vi "test_Task Actor1.vi"() -> ()   [LabVIEW 2023]
uses:
  <vilib>/ActorFramework/Actor/Actor.lvclass
  Task Actor/Task Actor.lvclass
  Task Base/Task Base.lvclass
  Measure and Stimulus Subsystems/Measure and Stimulus Subsystems.lvclass
  ITask Actor/ITask Actor Messages/Perform Action Msg/Perform Action Msg.lvclass
  <vilib>/ActorFramework/Stop Msg/Stop Msg.lvclass
  C:/Program Files/National Instruments/LabVIEW 2023/vi.lib/ActorFramework/Actor/Actor.lvclass
  D:/git/HAL/HAL GOOP4/Task Actor/Task Actor/Task Actor/Task Actor.lvclass
  D:/git/HAL/HAL GOOP4/Task Actor/ITask Actor/ITask Actor/ITask Actor.lvclass
panel:
  out "Waveform Graph Lossy":waveform(dbl)(graph)
  in  "Stop":bool
  in  "Perform Action":bool
  out "error out":errorcluster
  in  "Error in":errorcluster
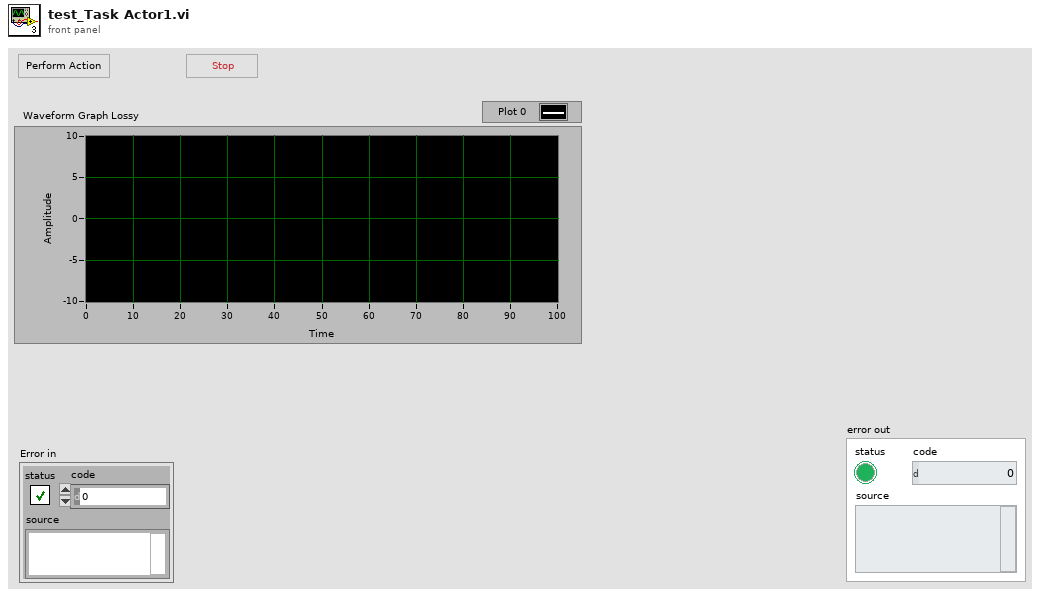
[diagram p1: front panel]
types:
  T1 = cluster{"Stop":refnum<notifier>, "Data":refnum<notifier>}
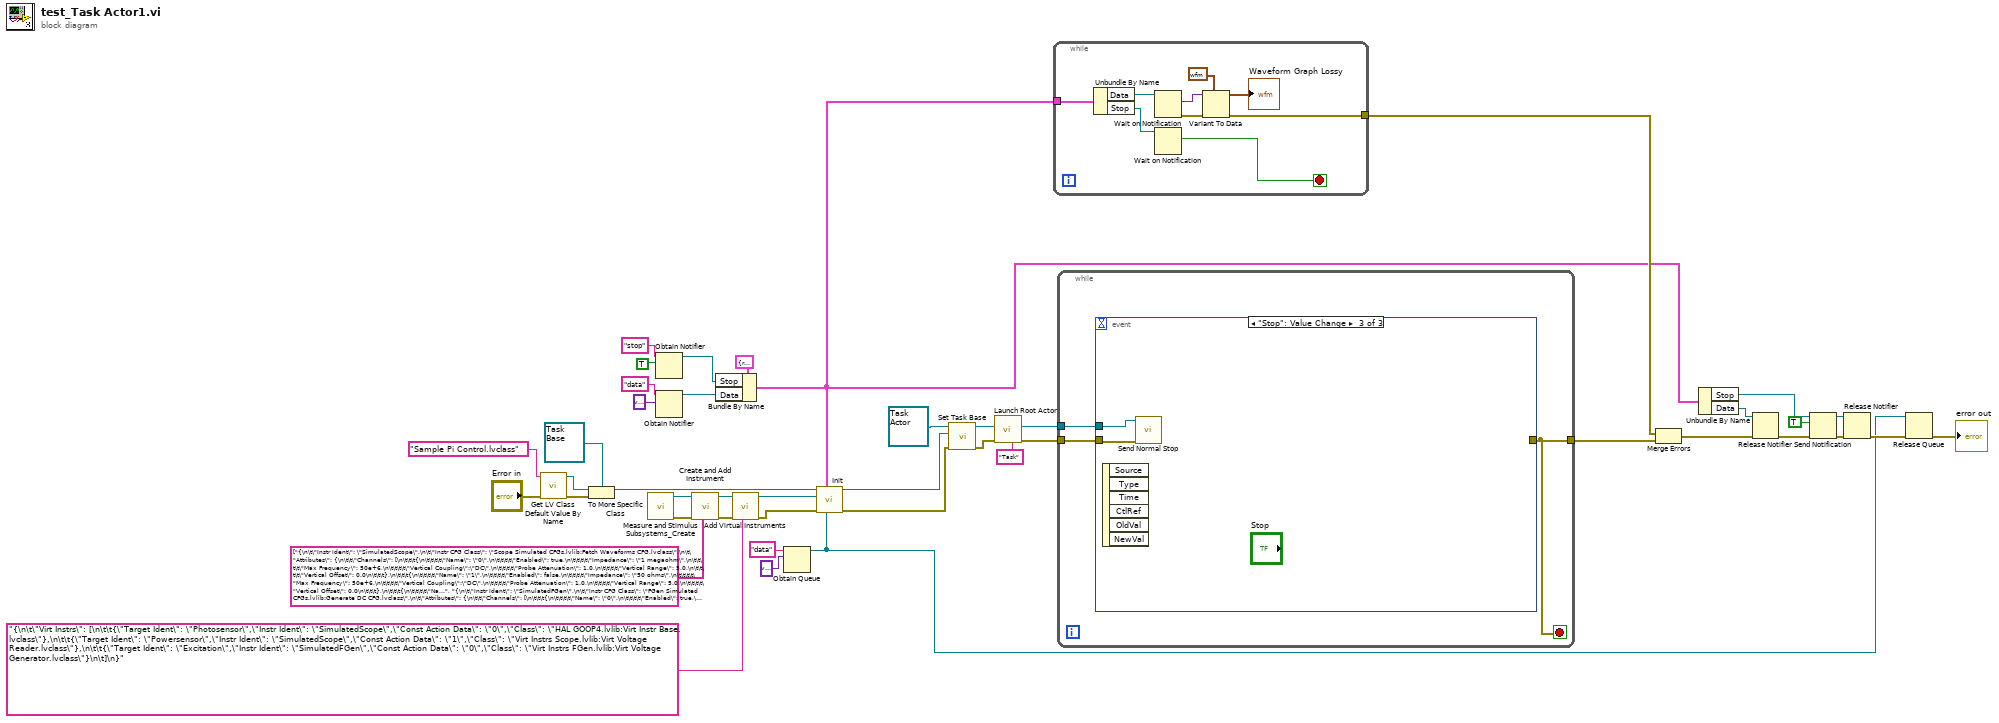
[diagram p0: block diagram]
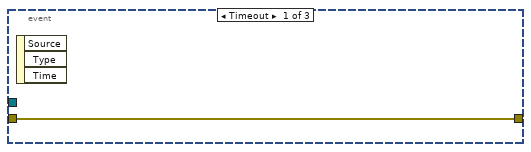
[diagram p2: hidden frame]
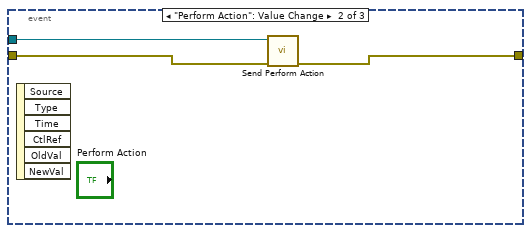
[diagram p3: hidden frame]
diagram:
  n1 = call <vilib>:"Get LV Class Default Value By Name.vi"("error in (no error)"="Error in", "class name"="Sample Pi Control.lvclass") -> ("error out"=w38:errorcluster, "object"=w39:refnum<class>)  [unwired: 8 in]
  n2 = To More Specific Class(target class=refnum<class "Task Base.lvclass"> refnum ("HAL GOOP4.lvlib:Task Base.lvclass"), reference=w39, error in=w38) -> (specific class reference=w36:refnum<class "Task Base.lvclass">)  [unwired: 1 out]
  n3 = call "Measure and Stimulus Subsystems_Create.vi"() -> ("Error Out"=w35:errorcluster, "reference out"=w28:refnum<class "Measure and Stimulus Subsystems.lvclass">)  [unwired: 10 in]
  n4 = Obtain Notifier(name (unnamed)="stop", notification data type=TRUE) -> (notifier out=w23:refnum<notifier>)  [unwired: 2 in, 2 out]
  n5 = Obtain Notifier(name (unnamed)="data", notification data type=variant) -> (notifier out=w22:refnum<notifier>)  [unwired: 2 in, 2 out]
  n6 = call "Create and Add Instrument.vi"("Physical Intr Configs"=string[] ["{\n\t\"Instr Ident\": \"SimulatedScope\",\n\t\"Instr CFG Class\": \"Scope Simulated CFGs.lvlib:Fetch Waveforms CFG.lvclass\",\n\t\"Attributes\": {\n\t\t\"Channels\": [\n\t\t\t{\n\t\t\t\t\"Name\": \"0\",\n\t\t\t\t\"Enabled\": true,\n\t\t\t\t\"Impedance\": \"1 megaohm\",\n\t\t\t\t\"Max Frequency\": 50e+6,\n\t\t\t\t\"Vertical Coupling\":\"DC\",\n\t\t\t\t\"Probe Attenuation\": 1.0,\n\t\t\t\t\"Vertical Range\": 5.0,\n\t\t\t\t\"Vertical Offset\": 0.0\n\t\t\t},\n\t\t\t{\n\t\t\t\t\"Name\": \"1\",\n\t\t\t\t\"Enabled\": false,\n\t\t\t\t\"Impedance\": \"50 ohms\",\n\t\t\t\t\"Max Frequency\": 50e+6,\n\t\t\t\t\"Vertical Coupling\":\"DC\",\n\t\t\t\t\"Probe Attenuation\": 1.0,\n\t\t\t\t\"Vertical Range\": 5.0,\n\t\t\t\t\"Vertical Offset\": 0.0\n\t\t\t},\n\t\t\t{\n\t\t\t\t\"Name\": \"2\",\n\t\t\t\t\"Enabled\": false,\n\t\t\t\t\"Impedance\": \"50 ohms\",\n\t\t\t\t\"Max Frequency\": 50e+6,\n\t\t\t\t\"Vertical Coupling\":\"DC\",\n\t\t\t\t\"Probe Attenuation\": 1.0,\n\t\t\t\t\"Vertical Range\": 5.0,\n\t\t\t\t\"Vertical Offset\": 0.0\n\t\t\t},\n\t\t\t{\n\t\t\t\t\"Name\": \"3\",\n\t\t\t\t\"Enabled\": true,\n\t\t\t\t\"Impedance\": \"50 ohms\",\n\t\t\t\t\"Max Frequency\": 50e+6,\n\t\t\t\t\"Vertical Coupling\":\"DC\",\n\t\t\t\t\"Probe Attenuation\": 1.0,\n\t\t\t\t\"Vertical Range\": 1.4,\n\t\t\t\t\"Vertical Offset\": 0.0\n\t\t\t},\n\t\t\t{\n\t\t\t\t\"Name\": \"4\",\n\t\t\t\t\"Enabled\": false,\n\t\t\t\t\"Impedance\": \"50 ohms\",\n\t\t\t\t\"Max Frequency\": 50e+6,\n\t\t\t\t\"Vertical Coupling\":\"DC\",\n\t\t\t\t\"Probe Attenuation\": 1.0,\n\t\t\t\t\"Vertical Range\": 5.0,\n\t\t\t\t\"Vertical Offset\": 0.0\n\t\t\t},\n\t\t\t{\n\t\t\t\t\"Name\": \"5\",\n\t\t\t\t\"Enabled\": false,\n\t\t\t\t\"Impedance\": \"50 ohms\",\n\t\t\t\t\"Max Frequency\": 50e+6,\n\t\t\t\t\"Vertical Coupling\":\"DC\",\n\t\t\t\t\"Probe Attenuation\": 1.0,\n\t\t\t\t\"Vertical Range\": 5.0,\n\t\t\t\t\"Vertical Offset\": 0.0\n\t\t\t},\n\t\t\t{\n\t\t\t\t\"Name\": \"6\",\n\t\t\t\t\"Enabled\": false,\n\t\t\t\t\"Impedance\": \"50 ohms\",\n\t\t\t\t\"Max Frequency\": 50e+6,\n\t\t\t\t\"Vertical Coupling\":\"DC\",\n\t\t\t\t\"Probe Attenuation\": 1.0,\n\t\t\t\t\"Vertical Range\": 5.0,\n\t\t\t\t\"Vertical Offset\": 0.0\n\t\t\t},\n\t\t\t{\n\t\t\t\t\"Name\": \"7\",\n\t\t\t\t\"Enabled\": false,\n\t\t\t\t\"Impedance\": \"50 ohms\",\n\t\t\t\t\"Max Frequency\": 50e+6,\n\t\t\t\t\"Vertical Coupling\":\"DC\",\n\t\t\t\t\"Probe Attenuation\": 1.0,\n\t\t\t\t\"Vertical Range\": 5.0,\n\t\t\t\t\"Vertical Offset\": 0.0\n\t\t\t}\n\t\t],\n\t\t\"Horizontal\": {\n\t\t\t\"Enforce Realtime\": true,\n\t\t\t\"Number of Records\": 1,\n\t\t\t\"Min Sample Rate\": 1e+5,\n\t\t\t\"Reference Position\":50, //percent\n\t\t\t\"Min Record Length\":1e+3\n\t\t},\n\t\t\"Acquire\": {\n\t\t\t\"Type\": \"Normal\",\n\t\t\t\"NumSamples\": 1e+3,\n\t\t\t\"Fetch Relative To\": \"Read Pointer\"\n\t\t},\n\t\t\"Export Signal\": {\n\t\t\t\"Signal Identifier\": \"None\",\n\t\t\t\"Signal\": \"None\",\n\t\t\t\"Output Terminal\": \"None\"\n\t\t},\n\t\t\"Trigger\": {\n\t\t\t\"Type\": \"Immediate\",\n\t\t\t\"Slope\": \"Positive\",\n\t\t\t\"Source\": \"RTSI 0\",\n\t\t\t\"Holdoff\": 0.0,\n\t\t\t\"Delay\": 0.0\n\t\t}\n\t}\n}", "{\n\t\"Instr Ident\": \"SimulatedFGen\",\n\t\"Instr CFG Class\": \"FGen Simulated CFGs.lvlib:Generate DC CFG.lvclass\",\n\t\"Attributes\": {\n\t\t\"Channels\": [\n\t\t\t{\n\t\t\t\t\"Name\": \"0\",\n\t\t\t\t\"Enabled\": true,\n\t\t\t\t\"Waveform\": \"DC\",\n\t\t\t\t\"Frequency\": 0, //DC\n\t\t\t\t\"Amplitude\": 0.0,\n\t\t\t\t\"Start Phase\": 0.0,\n\t\t\t\t\"DC Offset\": 0.0,\n\t\t\t\t\"Trigger Mode\": \"Single\"\n\t\t\t}\n\t\t],\n\t\t\"Export Signal\": {\n\t\t\t\"Enabled\": true,\n\t\t\t\"Output Terminal\": \"PFI 0\",\n\t\t\t\"Signal Identifier\": \"None\",\n\t\t\t\"Signal\": \"Start Trigger\"\n\t\t}\n\t}\n}"], "Error In"=w35, "reference in"=w28) -> ("Error Out"=w34:errorcluster, "reference out"=w29:refnum<class "Measure and Stimulus Subsystems.lvclass">)  [unwired: 7 in]
  n7 = Bundle By Name(cluster=T1 {"Stop"=refnum, "Data"=refnum} ("Notifiers"), "Stop"=w23, "Data"=w22) -> (w6:T1)
  n8 = call "Add Virtual Instruments.vi"("<JSON CFG>"="{\n\t\"Virt Instrs\": [\n\t\t{\"Target Ident\": \"Photosensor\",\"Instr Ident\": \"SimulatedScope\",\"Const Action Data\": \"0\",\"Class\": \"HAL GOOP4.lvlib:Virt Instr Base.lvclass\"},\n\t\t{\"Target Ident\": \"Powersensor\",\"Instr Ident\": \"SimulatedScope\",\"Const Action Data\": \"1\",\"Class\": \"Virt Instrs Scope.lvlib:Virt Voltage Reader.lvclass\"},\n\t\t{\"Target Ident\": \"Excitation\",\"Instr Ident\": \"SimulatedFGen\",\"Const Action Data\": \"0\",\"Class\": \"Virt Instrs FGen.lvlib:Virt Voltage Generator.lvclass\"}\n\t]\n}", "Error In"=w34, "reference in"=w29) -> ("Error Out"=w32:errorcluster, "reference out"=w33:refnum<class "Measure and Stimulus Subsystems.lvclass">)  [unwired: 7 in]
  n9 = Obtain Queue(name (unnamed)="data", element data type=variant) -> (queue out=w7:refnum<queue>)  [unwired: 3 in, 2 out]
  n10 = call-dynamic "Init.vi"("Data Queue"=w7, "Notifiers"=w6, "error in (no error)"=w32, "MSS"=w33, "Task Base in"=w36) -> ("error out"=w18:errorcluster, "Task Base out"=w42:refnum<class "Task Base.lvclass">)  [unwired: 5 in]
  n11 = call "Set Task Base.vi"("error in (no error)"=w18, "HAL GOOP4.lvlib:Task Base.lvclass"=w42, "Task Actor in"=refnum<class "Task Actor.lvclass"> refnum ("Task Actor.lvlib:Task Actor.lvclass")) -> ("error out"=w17:errorcluster, "Task Actor out"=w43:refnum<class "Task Actor.lvclass">)  [unwired: 7 in]
  n12 = call <vilib>:"Launch Root Actor.vi"("Debug Alias"="Task", "error in (no error)"=w17, "Actor"=w43) -> ("error out"=w15:errorcluster, "Actor's Enqueuer"=w16:refnum<class "Message Enqueuer.lvclass">)  [unwired: 7 in]
  n13 = while {
    tunnel: w6 -> [w53]
    tunnel: [w45] -> w11
    stop <- w50 stop-if-true
    n14 = Unbundle By Name(w53) -> ("Data"=w52:refnum<notifier>, "Stop"=w51:refnum<notifier>)
    n15 = Wait on Notification(notifier=w52) -> (notification=w48:variant, error out=w49:errorcluster)  [unwired: 3 in, 2 out]
    n16 = Wait on Notification(notifier=w51) -> (notification=w50:bool)  [unwired: 3 in, 3 out]
    n17 = Variant To Data(error in=w49, type=waveform(dbl) {"t0"=timestamp(0 s since 1904-01-01), "dt"=1.0, "Y"=[]} ("Waveform"), Variant=w48) -> (data=→"Waveform Graph Lossy":waveform(dbl), error out=w45:errorcluster)
  }
  n18 = while {
    tunnel: w16 -> [w56]
    tunnel: w15 -> [w55]
    tunnel: [w54] -> w13
    stop <- w54 stop-if-true
    n19 = event shown="[2] \"Stop\": Value Change" {
      selector: _ -> [_ _ _]
      dyn-events: _ -> [_ _ _]
      timeout: _ -> [_ _ _]
      tunnel: w56 -> [_ w60 w61]
      tunnel: w55 -> [w57 w59 w62]
      tunnel: [w57 w58 _] -> w54
      event Timeout {
        n20 = event-data() -> ()  [unwired: 1 in, 3 out]
      }
      event "Perform Action": Value Change {
        n21 = event-data() -> ()  [unwired: 1 in, 6 out]
        n22 = call "Send Perform Action.vi"("error in (no error)"=w59, "Message Enqueuer"=w60) -> ("error out"=w58:errorcluster)  [unwired: 8 in, 1 out]
      }
      event "Stop": Value Change {
        n23 = event-data() -> ()  [unwired: 1 in, 6 out]
        n24 = call <vilib>:"Send Normal Stop.vi"("error in (no error)"=w62, "Message Enqueuer"=w61) -> ()  [unwired: 9 in, 1 out]
      }
    }
  }
  n25 = Merge Errors(w11, w13) -> (w12:errorcluster)
  n26 = Unbundle By Name(w6) -> ("Stop"=w3:refnum<notifier>, "Data"=w5:refnum<notifier>)
  n27 = Release Notifier(notifier=w5, error in (no error)=w12) -> (error out=w10:errorcluster)  [unwired: 1 in, 2 out]
  n28 = Send Notification(notification=TRUE, notifier=w3, error in (no error)=w10) -> (notifier out=w2:refnum<notifier>, error out=w4:errorcluster)
  n29 = Release Notifier(notifier=w2, error in (no error)=w4) -> (error out=w9:errorcluster)  [unwired: 1 in, 2 out]
  n30 = Release Queue(queue=w7, error in (no error)=w9) -> (error out=→"error out":errorcluster)  [unwired: 1 in, 2 out]
